vi "Test HSE_v2 Format String.vi"(8 "error in (no error)":errorcluster) -> (0 "error out":errorcluster)   [LabVIEW 2016, in "UT_Formatter.lvlib"]
doc: "Template for an unit test with caraya in the \"Given, When, Then\" structure from James."
uses:
  UT_Formatter.lvlib
  Source/HSE-Logger/LogLevel.ctl
  Source/HSE-Logger/LogRecord/LogRecord.lvclass/LogRecord.ctl
  <vilib>/addons/_JKI Toolkits/Caraya/classes/Assert/Assert Equal Value_Variant.vi
  Source/HSE-Logger/Formatter/HSE_v2_Formatter/HSE_v2_Formatter.lvclass
  <vilib>/addons/_JKI Toolkits/Caraya/classes/Test/Test.lvclass
  <vilib>/addons/_JKI Toolkits/Caraya/classes/Assert/Assert.lvclass
  Source/HSE-Logger/LogRecord/LogRecord.lvclass
  Source/HSE-Logger/hse-logger.lvlib
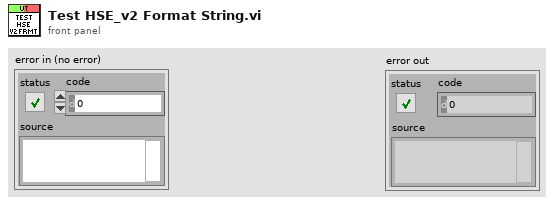
[diagram p1: front panel]
types:
  T1 = typedef "hse-logger.lvlib/LogLevel.ctl" = enum16{"DEBUG", "INFO", "WARNING", "ERROR", "CRITICAL"}
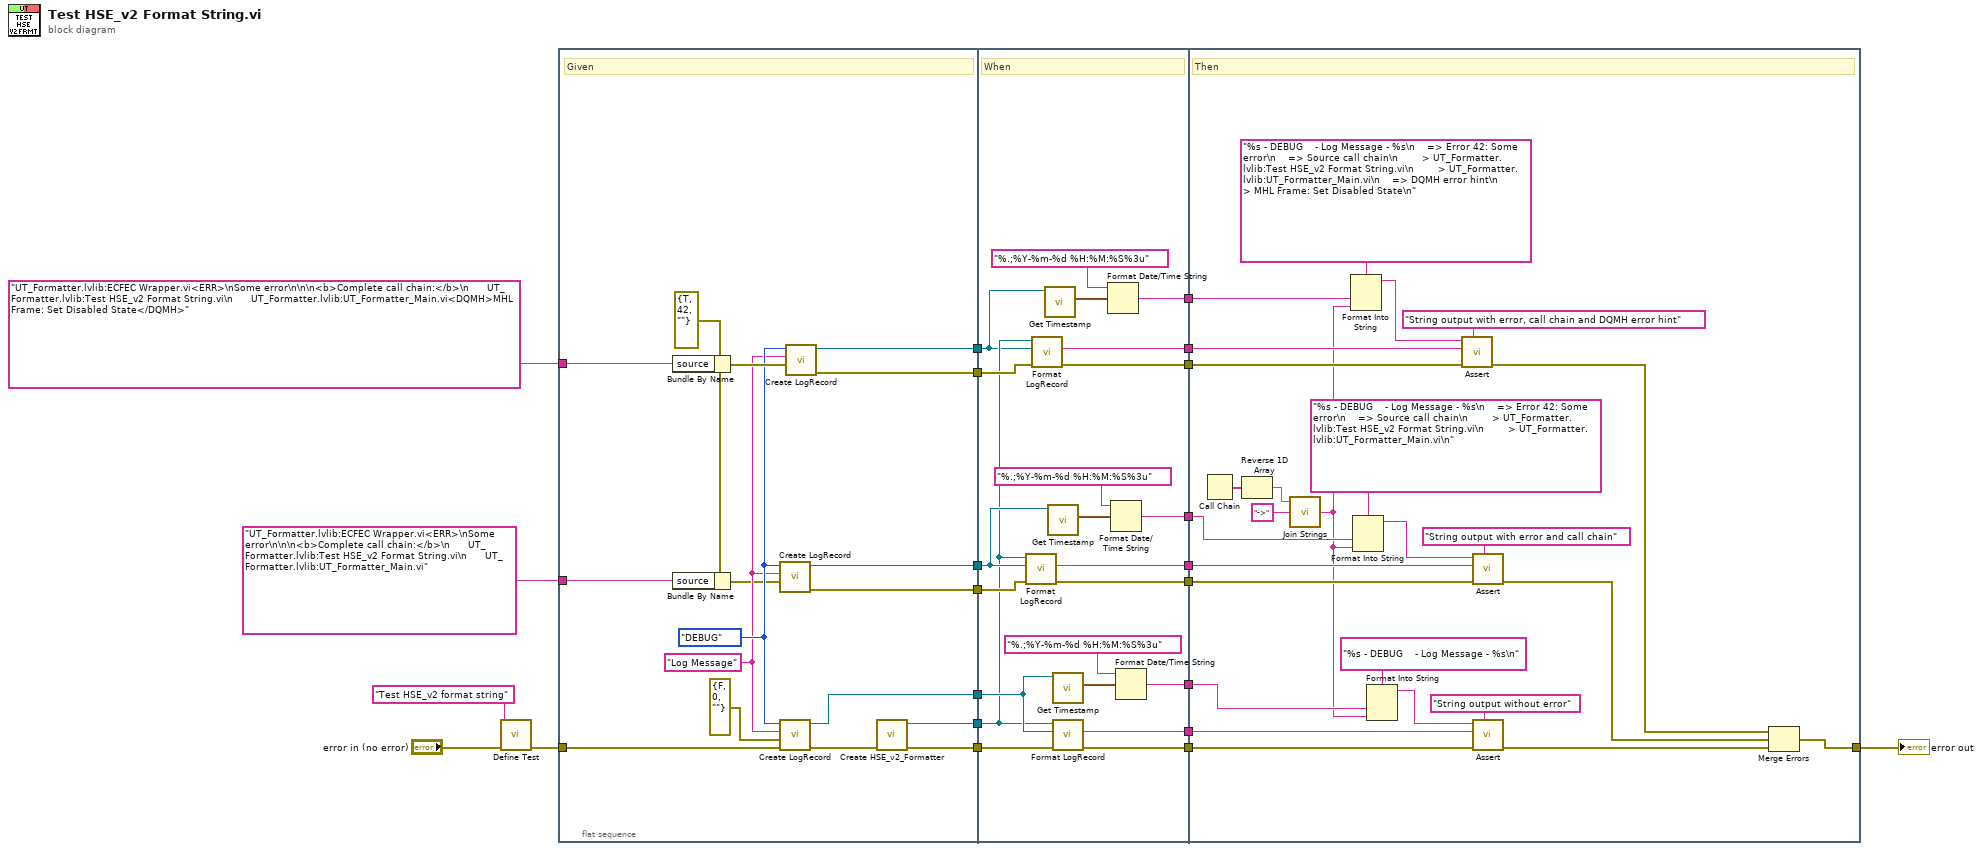
[diagram p0: block diagram]
diagram:
  n1 = call <vilib>:"Define Test.vi"("error in (no error)"="error in (no error)", "Label (VI Title)"="Test HSE_v2 format string") -> ("error out"=w19:errorcluster)  [unwired: 8 in, 1 out]
  n2 = flat-sequence {
    tunnel: w19 -> [w39]
    tunnel: [w33] -> w22
    tunnel: [w32] -> w16
    tunnel: [w37] -> w15
    tunnel: [w36] -> w12
    tunnel: [w35] -> w11
    tunnel: [w28] -> w7
    tunnel: [w27] -> w6
    tunnel: "UT_Formatter.lvlib:ECFEC Wrapper.vi<ERR>\nSome error\n\n\n<b>Complete call chain:</b>\n      UT_Formatter.lvlib:Test HSE_v2 Format String.vi\n      UT_Formatter.lvlib:UT_Formatter_Main.vi<DQMH>MHL Frame: Set Disabled State</DQMH>" ("source") -> [w24]
    tunnel: "UT_Formatter.lvlib:ECFEC Wrapper.vi<ERR>\nSome error\n\n\n<b>Complete call chain:</b>\n      UT_Formatter.lvlib:Test HSE_v2 Format String.vi\n      UT_Formatter.lvlib:UT_Formatter_Main.vi" ("source") -> [w23]
    tunnel: w22 -> [w61]
    tunnel: [w60] -> w17
    tunnel: w16 -> [w46]
    tunnel: w15 -> [w58]
    tunnel: [w59] -> w14
    tunnel: [w57] -> w13
    tunnel: w12 -> [w56]
    tunnel: w11 -> [w52]
    tunnel: [w55] -> w10
    tunnel: [w54] -> w9
    tunnel: [w51] -> w8
    tunnel: w7 -> [w47]
    tunnel: w6 -> [w44]
    tunnel: [w42] -> w5
    tunnel: [w41] -> w4
    tunnel: [w40] -> w1
    tunnel: [w87] -> w21
    tunnel: w17 -> [w85]
    tunnel: w14 -> [w83]
    tunnel: w13 -> [w80]
    tunnel: w10 -> [w78]
    tunnel: w9 -> [w79]
    tunnel: w8 -> [w76]
    tunnel: w5 -> [w69]
    tunnel: w4 -> [w64]
    tunnel: w1 -> [w63]
    frame #0 {
      w26 = errorcluster {"status"=TRUE, "code"=42, "source"=""} ("Error to Log")
      w29 = "Log Message" ("Message")
      w30 = LogLevel."DEBUG" ("Level")
      # "Given"
      n3 = Bundle By Name(cluster=w26, "source"=w24) -> (w31:errorcluster)
      n4 = Bundle By Name(cluster=w26, "source"=w23) -> (w25:errorcluster)
      n5 = call "Create LogRecord.vi"("Error to Log"=w25, "Message"=w29, "Level"=w30) -> ("error out"=w36:errorcluster, "LogRecord out"=w35:refnum<class "LogRecord.lvclass">)  [unwired: 7 in]
      n6 = call "Create LogRecord.vi"("error in"=w39, "Error to Log"=errorcluster {"status"=FALSE, "code"=0, "source"=""}, "Message"=w29, "Level"=w30) -> ("error out"=w34:errorcluster, "LogRecord out"=w37:refnum<class "LogRecord.lvclass">)  [unwired: 6 in]
      n7 = call "Create LogRecord.vi"("Error to Log"=w31, "Message"=w29, "Level"=w30) -> ("error out"=w28:errorcluster, "LogRecord out"=w27:refnum<class "LogRecord.lvclass">)  [unwired: 7 in]
      n8 = call "Create HSE_v2_Formatter.vi"("error in"=w34) -> ("error out"=w33:errorcluster, "HSE_v2_Formatter out"=w32:refnum<class "HSE_v2_Formatter.lvclass">)  [unwired: 9 in]
    }
    frame #1 {
      # "When"
      n9 = call-dynamic "Format LogRecord.vi"("error in"=w56, "LogRecord"=w52, "HSE_v2_Formatter in"=w46) -> ("error out"=w54:errorcluster, "LogLine"=w55:string)  [unwired: 7 in]
      n10 = call-dynamic "Format LogRecord.vi"("error in"=w47, "LogRecord"=w44, "HSE_v2_Formatter in"=w46) -> ("error out"=w42:errorcluster, "LogLine"=w41:string)  [unwired: 7 in]
      n11 = call "Get Timestamp.vi"("LogRecord in"=w44) -> ("Created"=w45:timestamp)  [unwired: 8 in, 2 out]
      n12 = call "Get Timestamp.vi"("LogRecord in"=w52) -> ("Created"=w53:timestamp)  [unwired: 8 in, 2 out]
      n13 = call "Get Timestamp.vi"("LogRecord in"=w58) -> ("Created"=w49:timestamp)  [unwired: 8 in, 2 out]
      n14 = call-dynamic "Format LogRecord.vi"("error in"=w61, "LogRecord"=w58, "HSE_v2_Formatter in"=w46) -> ("error out"=w60:errorcluster, "LogLine"=w59:string)  [unwired: 7 in]
      n15 = Format Date/Time String(time format string (%c)="%.;%Y-%m-%d %H:%M:%S%3u", seconds (now)=w45) -> (date/time string=w40:string)  [unwired: 1 in]
      n16 = Format Date/Time String(time format string (%c)="%.;%Y-%m-%d %H:%M:%S%3u", seconds (now)=w53) -> (date/time string=w51:string)  [unwired: 1 in]
      n17 = Format Date/Time String(time format string (%c)="%.;%Y-%m-%d %H:%M:%S%3u", seconds (now)=w49) -> (date/time string=w57:string)  [unwired: 1 in]
    }
    frame #2 {
      # "Then"
      n18 = Call Chain() -> (call chain=w71:string[])
      n19 = Reverse 1D Array(array=w71) -> (reversed array=w72:string[])
      n20 = call <vilib>:"Join Strings.vi"("Separator (,)"="->", "Strings In"=w72) -> ("String"=w62:string)  [unwired: 1 in]
      n21 = Format Into String(format string="%s - DEBUG    - Log Message - %s\n    => Error 42: Some error\n    => Source call chain\n        > UT_Formatter.lvlib:Test HSE_v2 Format String.vi\n        > UT_Formatter.lvlib:UT_Formatter_Main.vi\n    => DQMH error hint\n        > MHL Frame: Set Disabled State\n" ("Label"), w63, w62) -> (resulting string=w65:string)  [unwired: 2 in, 1 out]
      n22 = Format Into String(format string="%s - DEBUG    - Log Message - %s\n    => Error 42: Some error\n    => Source call chain\n        > UT_Formatter.lvlib:Test HSE_v2 Format String.vi\n        > UT_Formatter.lvlib:UT_Formatter_Main.vi\n" ("Label"), w76, w62) -> (resulting string=w74:string)  [unwired: 2 in, 1 out]
      n23 = Format Into String(format string="%s - DEBUG    - Log Message - %s\n" ("Label"), w80, w62) -> (resulting string=w82:string)  [unwired: 2 in, 1 out]
      n24 = call-poly <vilib>:"Assert.vi"("Label"="String output with error, call chain and DQMH error hint", "error in (no error)"=w69, "Y"=w64, "X"=w65) -> ("error out"=w68:errorcluster)  [unwired: 6 in, 1 out]
      n25 = call-poly <vilib>:"Assert.vi"("Label"="String output with error and call chain", "error in (no error)"=w79, "Y"=w78, "X"=w74) -> ("error out"=w73:errorcluster)  [unwired: 6 in, 1 out]
      n26 = call-poly <vilib>:"Assert.vi"("Label"="String output without error", "error in (no error)"=w85, "Y"=w83, "X"=w82) -> ("error out"=w84:errorcluster)  [unwired: 6 in, 1 out]
      n27 = Merge Errors(w68, w73, w84) -> (w87:errorcluster)
    }
  }
  "error out" <- w21
